vi "Get Default Config Path.vi"(8 "error in (no error)":errorcluster) -> (0 "error out":errorcluster, 3 "appended path":path)   [LabVIEW 2020, in "Base.lvclass"]
doc: "Generates the default configuration path. \nWhen called from the development environement, the default config path is the /Config relative to the project path.\nWhen called from a built exe the default config path is at C:\\Users\\<username>\\AppData\\Local\\<CompanyName>\\<ProductName> where company name and product name are the ones configured in the build specification.\nOn Linux the default config directory is \\home\\lvuser\\natinst\\bin\\config."
uses:
  Base.lvclass
  <vilib>/Utility/sysdir.llb/System Directory Type.ctl
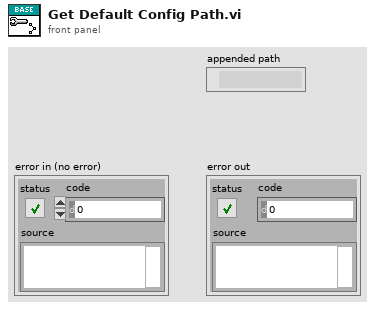
[diagram p1: front panel]
types:
  T1 = typedef "System Directory Type.ctl" = i32
  T2 = typedef "FileVersionInformation.ctl" = cluster{"FileVersion":string, "ProductName":string, "InternalName":string, "CompanyName":string, "LegalCopyright":string, "FileDescription":string}
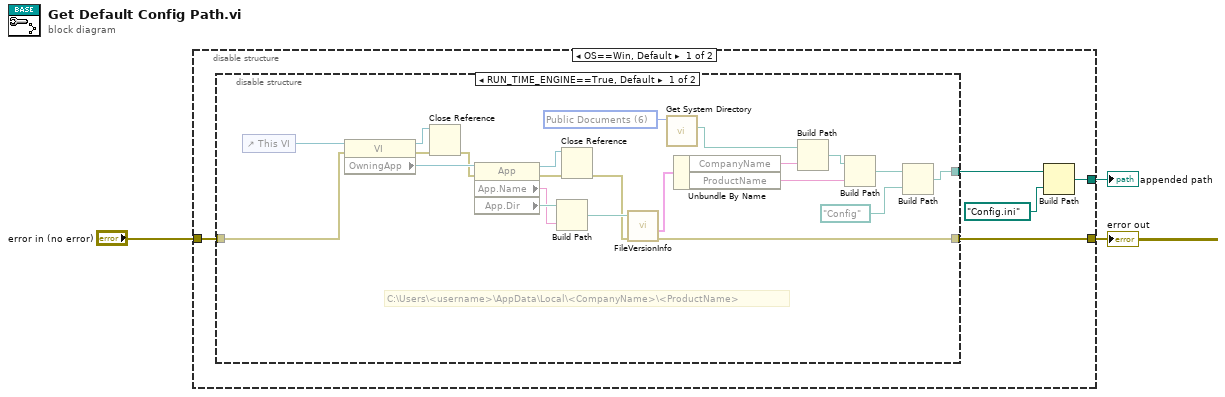
[diagram p0: block diagram]
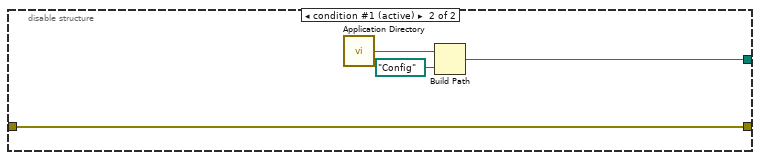
[diagram p2: hidden frame]
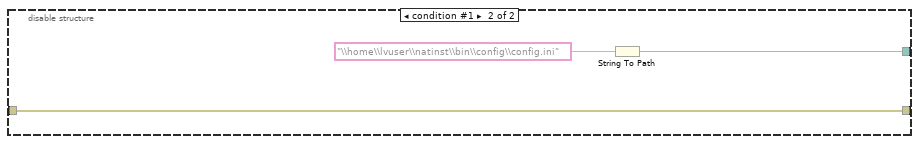
[diagram p3: hidden frame]
diagram:
  n1 = disable-structure shown="OS==Win, Default" {
    disable-tunnel: "error in (no error)" -> [w8 w37]
    disable-tunnel: [w7 w37] -> w3
    disable-tunnel: [w5 w36] -> w1
    frame condition #0 (active) {
      n2 = disable-structure shown="RUN_TIME_ENGINE==True, Default" {
        disable-tunnel: w8 -> [w20 w31]
        disable-tunnel: [w19 w31] -> w7
        disable-tunnel: [w11 w32] -> w6
        frame condition #0 {
          w18 = T1 6 items=["User Home"=0, "User Desktop"=1, "User Documents"=2, "User Application Data"=3, "User Preferences"=4, "User Temporary"=5, "Public Documents"=6, "Public Application Data"=7, "Public Preferences"=8, "Public Cache"=13, "System Core Libraries"=9, "System Installed Libraries"=10, "Application Files"=11, "Boot Volume Root"=12] ("system directory type")
          # "C:\\Users\\<username>\\AppData\\Local\\<CompanyName>\\<ProductName>"
          n3 = control-ref of="This VI"() -> (w12:refnum<vi>)
          n4 = property class="VI"(reference=w12, error in=w20) -> (reference out=w23:refnum<vi>, error out=w25:errorcluster, "OwningApp"=w30:refnum<vi>)
          n5 = Close Reference(reference=w23, error in (no error)=w25) -> (error out=w24:errorcluster)
          n6 = property class="App"(reference=w30, error in=w24) -> (reference out=w21:refnum<vi>, error out=w26:errorcluster, "App.Name"=w28:string, "App.Dir"=w29:path)
          n7 = Build Path(base path=w29, name or relative path=w28) -> (appended path=w27:path)
          n8 = Close Reference(reference=w21, error in (no error)=w26) -> (error out=w22:errorcluster)
          n9 = call <vilib>:"FileVersionInfo.vi"("error in (no error)"=w22, "Application Path in"=w27) -> ("error out"=w19:errorcluster, "FileVersionInfo Out"=w17:T2)  [unwired: 6 in, 2 out]
          n10 = call <vilib>:"Get System Directory.vi"("system directory type"=w18) -> ("system directory"=w13:path)  [unwired: 10 in]
          n11 = Unbundle By Name(w17) -> ("CompanyName"=w14:string, "ProductName"=w16:string)
          n12 = Build Path(base path=w13, name or relative path=w14) -> (appended path=w15:path)
          n13 = Build Path(base path=w15, name or relative path=w16) -> (appended path=w10:path)
          n14 = Build Path(base path=w10, name or relative path=path "Config") -> (appended path=w11:path)
        }
        frame condition #1 (active) {
          n15 = call <vilib>:"Application Directory.vi"() -> ("Application Directory"=w34:path)
          n16 = Build Path(base path=w34, name or relative path=path "Config") -> (appended path=w32:path)
        }
      }
      n17 = Build Path(base path=w6, name or relative path=path "Config.ini") -> (appended path=w5:path)
    }
    frame condition #1 {
      n18 = String To Path(string="\\home\\lvuser\\natinst\\bin\\config\\config.ini") -> (path=w36:path)
    }
  }
  "appended path" <- w1
  "error out" <- w3
